vi "Get Internal Command Data References.vi"(8 "error in (no error)":errorcluster, 11 "Addon Ref in":T1 format="%.0x") -> (0 "error out":errorcluster, 1 "VS Ref Groups":T2(array[cluster]) {"VS Refs" format="%.0x"}, 3 "Addon Ref out":T1 format="%.0x")   [LabVIEW 2019, in "J1939 Addon System Explorer.lvlib"]
uses:
  J1939 Addon System Explorer.lvlib
  <vilib>/NI VeriStand/Custom Device API/Custom Device Item Ref.ctl
  Addon Shared/SubVIs/Constants.vi
  <vilib>/NI VeriStand/Custom Device Tools/Custom Device Utility Library/NI VeriStand - Search for Item by Name.vi
  <vilib>/NI VeriStand/Custom Device Tools/Custom Device Utility Library/Custom Device Utility Library.lvlib
  Addon Shared/J1939 Addon Shared.lvlib
  <vilib>/NI VeriStand/Custom Device API/Custom Device API.lvlib
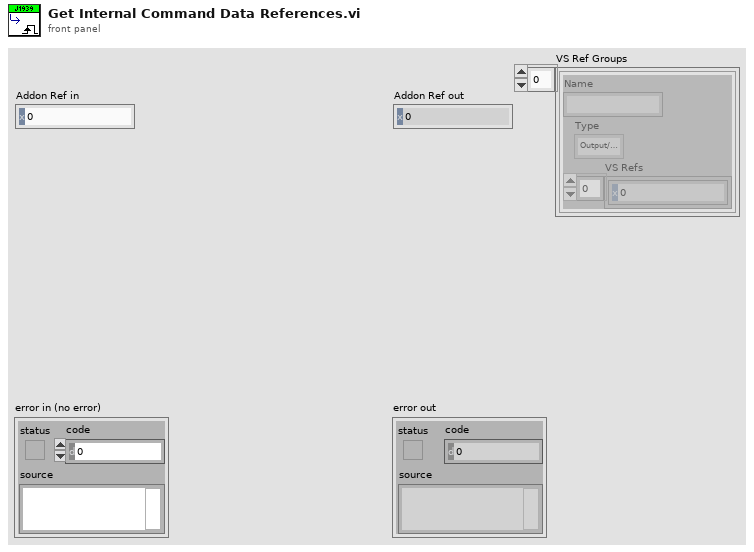
[diagram p1: front panel]
types:
  T1 = typedef "Custom Device API.lvlib/Custom Device Item Ref.ctl" = u64
  T2 = cluster{"Name":string, "Type":enum16{"Output/Write", "Input/Read", "Input/ReadWrite"}, "VS Refs":T1[]}[]
  T3 = enum16{"Output/Write", "Input/Read", "Input/ReadWrite"}
  T4 = cluster{"Name":string, "Type":enum16{"Output/Write", "Input/Read", "Input/ReadWrite"}, "VS Refs":T1[]}
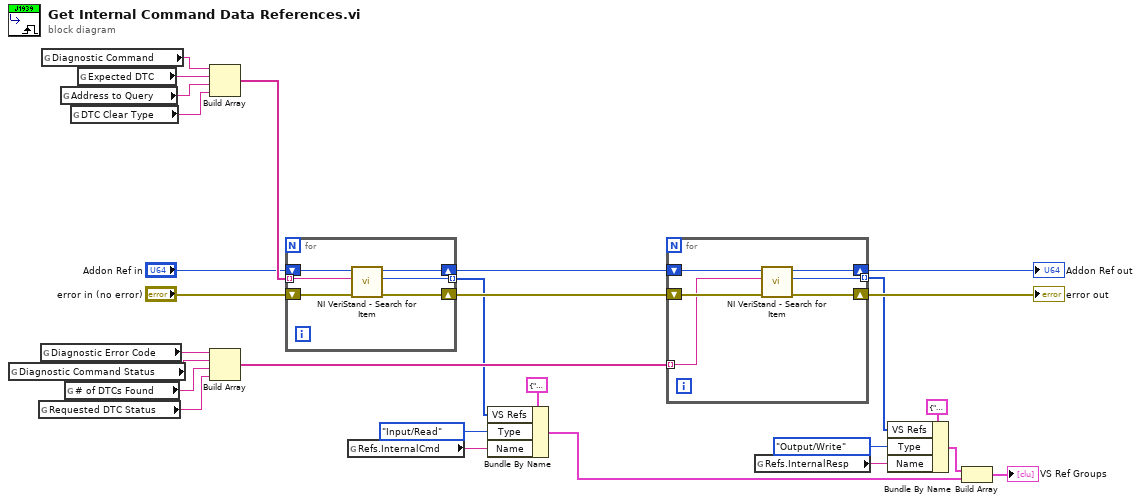
[diagram p0: block diagram]
diagram:
  n1 = global read "Constants.vi" "Diagnostic Command Status"() -> (w21:string)
  n2 = global read "Constants.vi" "Requested DTC Status"() -> (w23:string)
  n3 = global read "Constants.vi" "Diagnostic Error Code"() -> (w20:string)
  n4 = global read "Constants.vi" "Diagnostic Command"() -> (w27:string)
  n5 = global read "Constants.vi" "Address to Query"() -> (w25:string)
  n6 = global read "Constants.vi" "# of DTCs Found"() -> (w22:string)
  n7 = global read "Constants.vi" "DTC Clear Type"() -> (w24:string)
  n8 = global read "Constants.vi" "Expected DTC"() -> (w26:string)
  n9 = Build Array(w27, w26, w25, w24) -> (w19:string[])
  n10 = Build Array(w20, w21, w22, w23) -> (w18:string[])
  n11 = for {
    tunnel: [w33] -> w9 mode=indexing
    tunnel: w19 -> [w28] mode=indexing
    shift-right: [w31] -> w17
    shift-left: "error in (no error)" -> [w32]
    shift-right: [w30] -> w14
    shift-left: "Addon Ref in" -> [w29]
    n12 = call-poly <vilib>:"NI VeriStand - Search for Item.vi"("error in"=w32, "Item Name"=w28, "Section Ref in"=w29) -> ("error out"=w31:errorcluster, "Item Ref"=w33:T1, "Section Ref out"=w30:T1)  [unwired: 5 in, 1 out]
  }
  n13 = global read "Constants.vi" "Refs.InternalCmd"() -> (w12:string)
  n14 = Bundle By Name(cluster=T4 {"Name"="", "Type"=enum."Output/Write", "VS Refs"=[]} ("Group"), "VS Refs"=w9, "Type"=T3."Input/Read", "Name"=w12) -> (w2:T4)
  n15 = for {
    tunnel: [w38] -> w7 mode=indexing
    tunnel: w18 -> [w34] mode=indexing
    shift-right: [w36] -> w16
    shift-left: w17 -> [w37]
    shift-right: [w35] -> w15
    shift-left: w14 -> [w39]
    n16 = call-poly <vilib>:"NI VeriStand - Search for Item.vi"("error in"=w37, "Item Name"=w34, "Section Ref in"=w39) -> ("error out"=w36:errorcluster, "Item Ref"=w38:T1, "Section Ref out"=w35:T1)  [unwired: 5 in, 1 out]
  }
  "Addon Ref out" <- w15
  "error out" <- w16
  n17 = global read "Constants.vi" "Refs.InternalResp"() -> (w11:string)
  n18 = Bundle By Name(cluster=T4 {"Name"="", "Type"=enum."Output/Write", "VS Refs"=[]} ("Group"), "VS Refs"=w7, "Type"=T3."Output/Write", "Name"=w11) -> (w3:T4)
  n19 = Build Array(w3, w2) -> (→"VS Ref Groups":T2)
